vi "VISA Configure Serial Port - Rev A.vi"(0 "VISA resource name":refnum<visa-resource-name>, 1 "timeout (10sec)":u32=10000, 2 "termination char\n(0xA = '\\n' = LF)":u8=10 format="%.0x", 3 "Enable Termination\nChar (T)":bool=TRUE, 5 "baud rate (9600)":u32=9600, 7 "data bits (8)":u16=8 min=5 max=8 step=1, 9 "parity (0:none)":enum16{"None", "Odd", "Even", "Mark", "Space"}(ring), 11 "error in (no error)":errorcluster, 12 "stop bits (10: 1 bit)":u16(ring)=10 items=["1.0"=10, "1.5"=15, "2.0"=20], 13 "flow control (0:none)":u16(ring) items=["None", "XON/XOFF", "RTS/CTS", "XON/XOFF & RTS/CTS", "DTR/DSR", "XON/XOFF & DTR/DSR"]) -> (4 "VISA resource name out":refnum<visa-resource-name>, 15 "error out":errorcluster)   [LabVIEW 2017]
doc: "Initializes the serial port specified by <B>VISA resource name</B> to the specified settings. Wire data to the <B>VISA resource name</B> input to determine the polymorphic instance to use or manually select the instance."
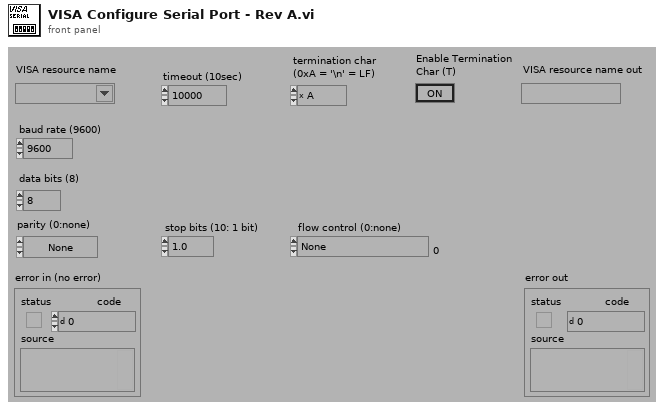
[diagram p1: front panel]
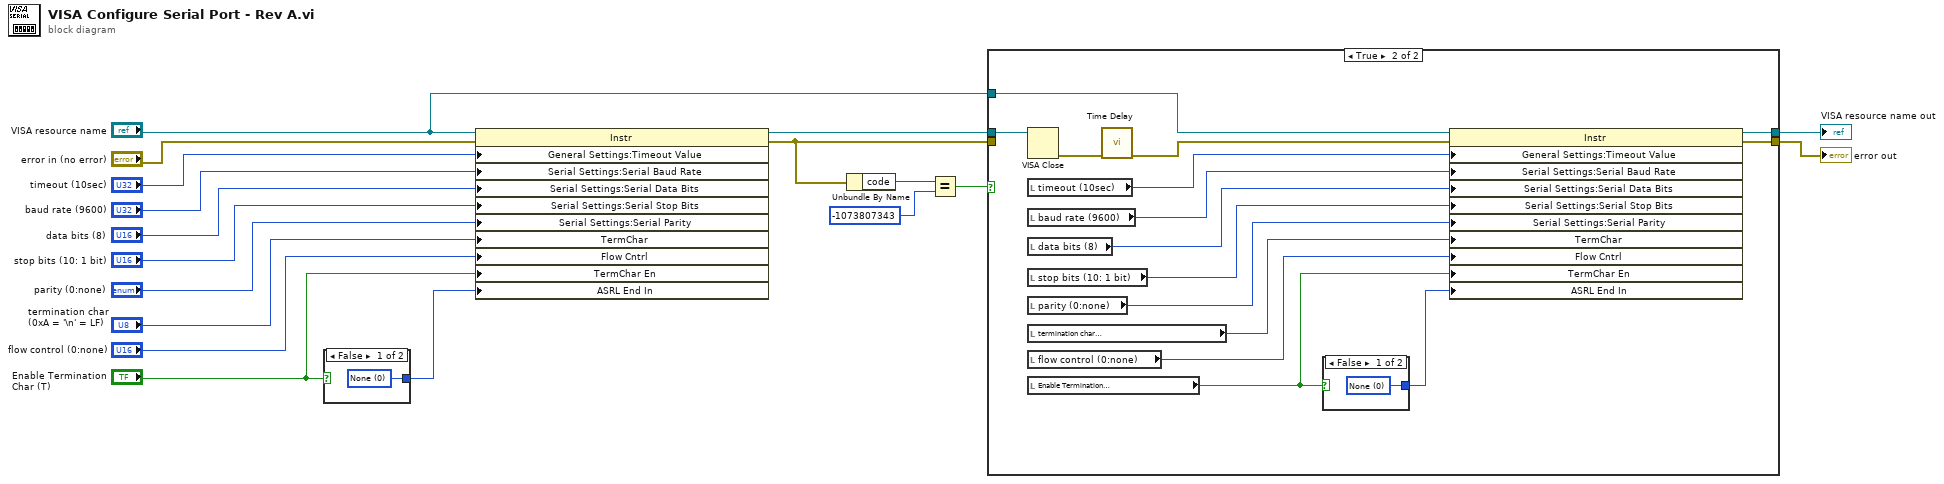
[diagram p0: block diagram]
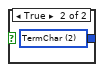
[diagram p3: hidden frame]
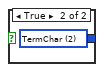
[diagram p4: hidden frame]
diagram:
  n1 = case shown="False" "Enable Termination\nChar (T)" {
    tunnel: [w19 w20] -> w9
    frame False {
      w19 = u16 0 items=["None", "LastBit", "TermChar"] ("Serial Settings:Serial End Mode for Reads")
    }
    frame True {
      w20 = u16 2 items=["None", "LastBit", "TermChar"] ("Serial Settings:Serial End Mode for Reads")
    }
  }
  n2 = property class="Instr"(reference="VISA resource name", error in="error in (no error)", "General Settings:Timeout Value"="timeout (10sec)", "Serial Settings:Serial Baud Rate"="baud rate (9600)", "Serial Settings:Serial Data Bits"="data bits (8)", "Serial Settings:Serial Stop Bits"="stop bits (10: 1 bit)", "Serial Settings:Serial Parity"="parity (0:none)", "TermChar"="termination char\n(0xA = '\\n' = LF)", "Flow Cntrl"="flow control (0:none)", "TermChar En"="Enable Termination\nChar (T)", "ASRL End In"=w9) -> (reference out=w5:refnum<visa-resource-name>, error out=w1:errorcluster)
  n3 = Unbundle By Name(w1) -> ("code"=w8:i32)
  n4 = Equal?(x=w8, y=-1073807343) -> (x = y?=w6:bool)
  n5 = case shown="True" w6 {
    tunnel: w5 -> [w22 w37]
    tunnel: "VISA resource name" -> [_ w35]
    tunnel: [w22 w24] -> w3
    tunnel: [w21 w23] -> w2
    tunnel: w1 -> [w21 _]
    frame False {
    }
    frame True {
      n6 = VISA Close(VISA resource name=w37) -> (error out=w36:errorcluster)  [unwired: 1 in]
      n7 = local read "timeout (10sec)"() -> (w33:u32)
      n8 = local read "baud rate (9600)"() -> (w32:u32)
      n9 = local read "data bits (8)"() -> (w31:u16)
      n10 = local read "stop bits (10: 1 bit)"() -> (w30:u16)
      n11 = local read "parity (0:none)"() -> (w29:enum16{"None", "Odd", "Even", "Mark", "Space"})
      n12 = local read "termination char\n(0xA = '\\n' = LF)"() -> (w28:u8)
      n13 = local read "flow control (0:none)"() -> (w27:u16)
      n14 = local read "Enable Termination\nChar (T)"() -> (w26:bool)
      n15 = call "Time Delay"("error in (no error)"=w36) -> ("error out"=w34:errorcluster)  [unwired: 10 in]
      n16 = case shown="False" w26 {
        tunnel: [w38 w39] -> w25
        frame False {
          w38 = u16 0 items=["None", "LastBit", "TermChar"] ("Serial Settings:Serial End Mode for Reads")
        }
        frame True {
          w39 = u16 2 items=["None", "LastBit", "TermChar"] ("Serial Settings:Serial End Mode for Reads")
        }
      }
      n17 = property class="Instr"(reference=w35, error in=w34, "General Settings:Timeout Value"=w33, "Serial Settings:Serial Baud Rate"=w32, "Serial Settings:Serial Data Bits"=w31, "Serial Settings:Serial Stop Bits"=w30, "Serial Settings:Serial Parity"=w29, "TermChar"=w28, "Flow Cntrl"=w27, "TermChar En"=w26, "ASRL End In"=w25) -> (reference out=w24:refnum<visa-resource-name>, error out=w23:errorcluster)
    }
  }
  "error out" <- w2
  "VISA resource name out" <- w3
